vi "check memory limit.vi"(8 "error in (no error)":errorcluster caption="에러 입력(에러 없음)", 10 "bytes of waveform":i32[](array[numeric]), 11 "DW7802 입력":refnum<class "DW7802.lvclass">) -> (0 "error out":errorcluster caption="에러 출력", 1 "message":string, 2 "disable?":T1(ring), 3 "DW7802 출력":refnum<class "DW7802.lvclass">)   [LabVIEW 2020, in "DW7802.lvclass"]
uses:
  DW7802.lvclass
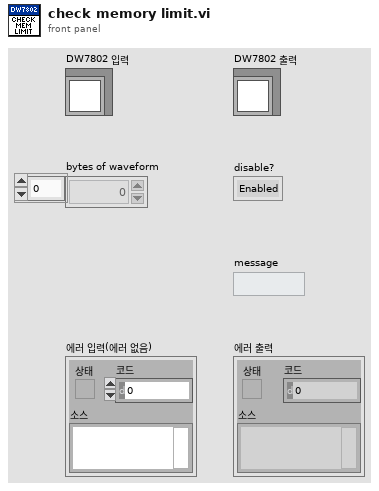
[diagram p1: front panel]
types:
  T1 = enum8{"Enabled", "Disabled", "Disabled and Grayed Out"}
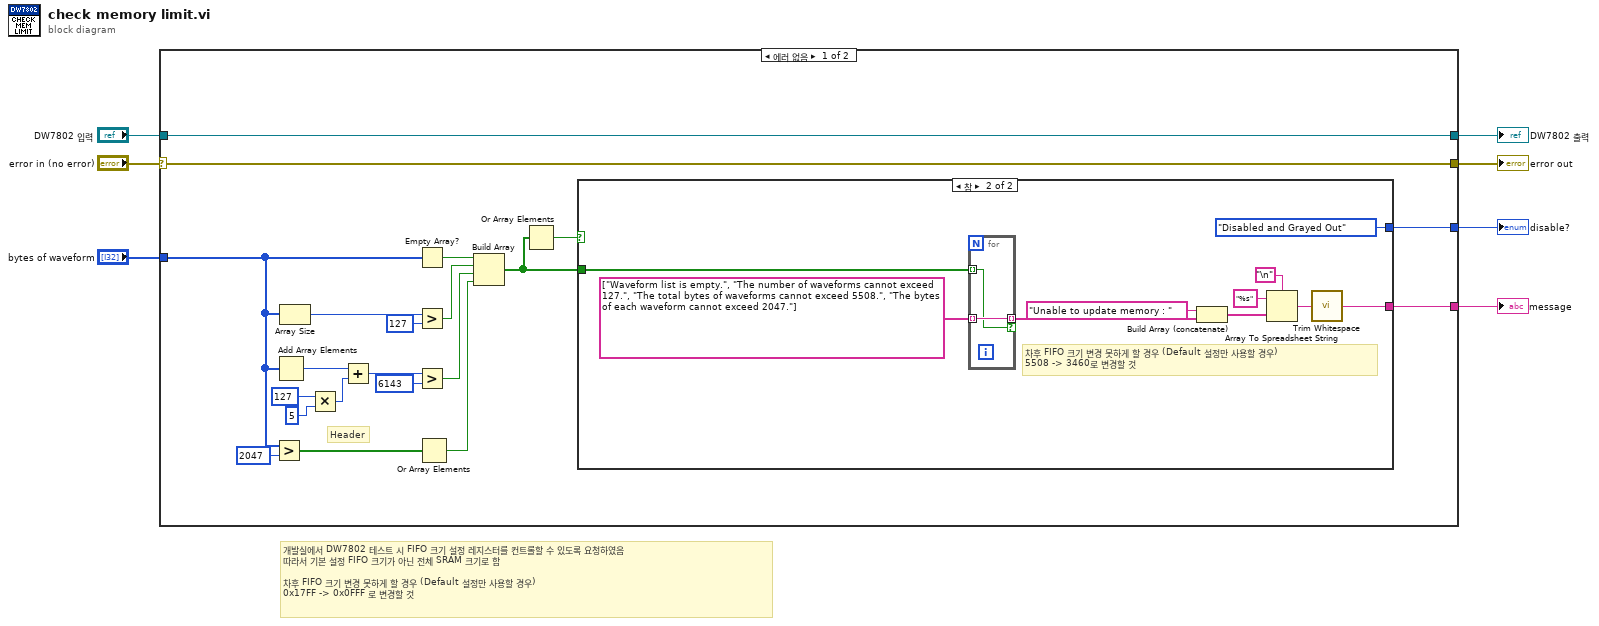
[diagram p0: block diagram]
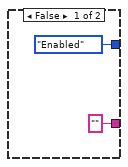
[diagram p2: hidden frame]
diagram:
  # "개발실에서 DW7802 테스트 시 FIFO 크기 설정 레지스터를 컨트롤할 수 있도록 요청하였음\n따라서 기본 설정 FIFO 크기가 아닌 전체 SRAM 크기로 함\n\n차후 FIFO 크기 변경 못하게 할 경우 (Default 설정만 사용할 경우) \n0x17FF -> 0x0FFF 로 변경할 것"
  n1 = case shown="에러 없음" "error in (no error)" {
    selector: "error in (no error)" -> [w28 w44]
    tunnel: [w28 w44] -> w7
    tunnel: "DW7802 입력" -> [w27 w43]
    tunnel: [w27 w43] -> w4
    tunnel: "bytes of waveform" -> [w19 _]
    tunnel: [w9 _] -> w6
    tunnel: [w8 _] -> w5
    frame No Error {
      # "Header"
      n2 = Greater?(x=w19, y=2047) -> (0:w20:bool[])
      n3 = Add Array Elements(numeric array=w19) -> (sum=w23:i32)
      n4 = Array Size(array=w19) -> (size(s)=w26:i32)
      n5 = Multiply(x=127, y=5) -> (x*y=w13:i32)
      n6 = Add(x=w23, y=w13) -> (x+y=w14:i32)
      n7 = Empty Array?(array=w19) -> (empty?=w18:bool)
      n8 = Greater?(x=w26, y=127) -> (0:w17:bool)
      n9 = Greater?(x=w14, y=6143) -> (0:w16:bool)
      n10 = Or Array Elements(Boolean array=w20) -> (logical OR=w15:bool)
      n11 = Build Array(w18, w17, w16, w15) -> (w11:bool[])
      n12 = Or Array Elements(Boolean array=w11) -> (logical OR=w10:bool)
      n13 = case shown="참" w10 {
        tunnel: w11 -> [_ w39]
        tunnel: ["" ("trimmed string") w32] -> w9
        tunnel: [T1."Enabled" ("disable?") T1."Disabled and Grayed Out" ("disable?")] -> w8
        frame False {
        }
        frame True {
          # "차후 FIFO 크기 변경 못하게 할 경우 (Default 설정만 사용할 경우)\n5508 -> 3460로 변경할 것"
          n14 = for {
            tunnel: w39 -> [w41] mode=indexing
            tunnel: string[] ["Waveform list is empty.", "The number of waveforms cannot exceed 127.", "The total bytes of waveforms cannot exceed 5508.", "The bytes of each waveform cannot exceed 2047."] -> [w42] mode=indexing
            tunnel: [w42] -> w38 mode=indexing if=w41
          }
          n15 = Build Array (concatenate)("Unable to update memory : " ("원소"), w38) -> (w33:string[])
          n16 = Array To Spreadsheet String(delimiter (Tab)="\n", array=w33, 3:"%s" ("포맷 문자열")) -> (spreadsheet string=w35:string)
          n17 = call <vilib>:"Trim Whitespace.vi"("string"=w35) -> ("trimmed string"=w32:string)  [unwired: 1 in]
        }
      }
    }
    frame Error {
    }
  }
  "error out" <- w7
  "DW7802 출력" <- w4
  "disable?" <- w5
  "message" <- w6
